vi "start.vi"(8 "error in (no error)":errorcluster, 11 "CQT_DDS in":refnum<class "CQT_DDS.lvclass">) -> (0 "error out":errorcluster, 3 "CQT_DDS out":refnum<class "CQT_DDS.lvclass">)   [LabVIEW 2009, in "Hardware.lvlib" / "Channels.lvlib" / "CQT_DDS.lvclass"]
uses:
  CQT_DDS.lvclass
  Generic/DDSOutput.lvclass
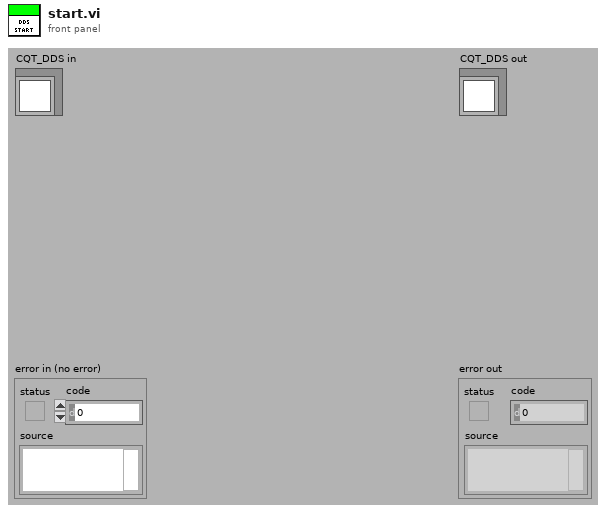
[diagram p1: front panel]
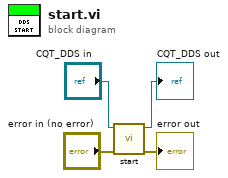
[diagram p0: block diagram]
diagram:
  n1 = call-parent "start.vi"("error in (no error)"="error in (no error)", "DDSOutput in"="CQT_DDS in") -> ("error out"=→"error out":errorcluster, "DDSOutput out"=→"CQT_DDS out":refnum<class "CQT_DDS.lvclass">)  [unwired: 8 in]
